vi "UDP Thread Settings UI.vi"(8 "error in (no error)":errorcluster, 10 "User Interface Events":refnum<class "User Interface Events.lvclass">, 11 "Configuration in":refnum<class "Configuration.lvclass">) -> (0 "error out":errorcluster, 3 "Configuration out":refnum<class "Configuration.lvclass">)   [LabVIEW 2017, in "DSF Core.lvlib"]
uses:
  DSF Core.lvlib
  Classes/Configuration/Configuration.lvclass
  Classes/User Interface Events/User Interface Events.lvclass
  Configuration/DSF UDP Thread Settings.lvclass
  C:/Git/DSF/Core/Classes/Configuration/Configuration.lvclass
panel:
  in  "local port":u16
  in  "local address":string
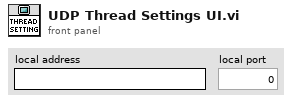
[diagram p1: front panel]
types:
  T1 = typedef "DSF Core.lvlib/DSF UDP Thread Settings.lvclass/Thread Settings.ctl" = cluster{"local port":u16, "local address":u32}
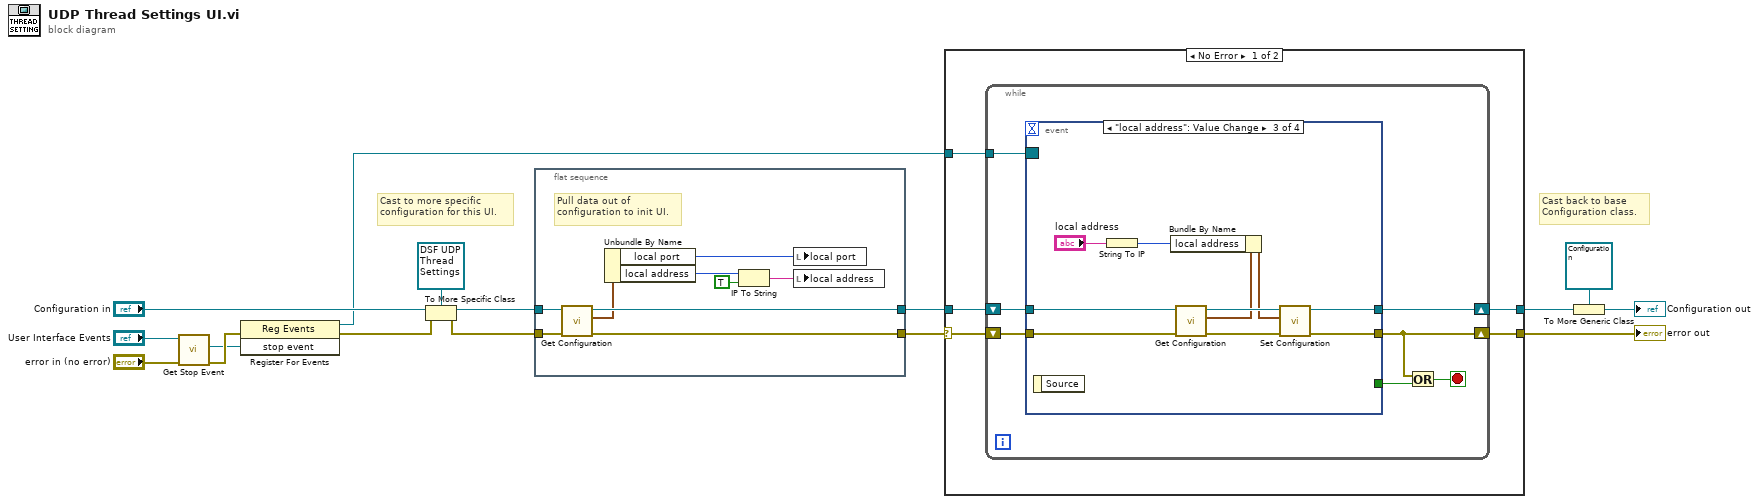
[diagram p0: block diagram]
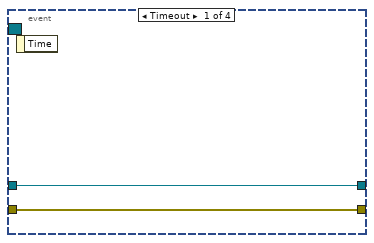
[diagram p2: hidden frame]
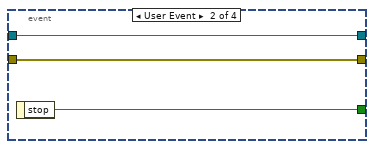
[diagram p3: hidden frame]
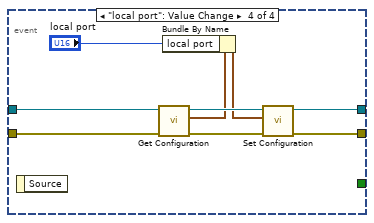
[diagram p4: hidden frame]
diagram:
  # "Cast back to base Configuration class."
  # "Cast to more specific configuration for this UI."
  n1 = call "Get Stop Event.vi"("error in (no error)"="error in (no error)", "User Interface Events in"="User Interface Events") -> ("error out"=w5:errorcluster, "stop event"=w3:refnum<user-event>)  [unwired: 7 in, 1 out]
  n2 = register-events(error in=w5, w3) -> (reference out=w6:refnum<event-registration>, error out=w7:errorcluster)  [unwired: 1 in]
  n3 = To More Specific Class(target class=refnum<class "DSF UDP Thread Settings.lvclass"> refnum ("DSF Core.lvlib:DSF UDP Thread Configuration"), reference="Configuration in", error in=w7) -> (specific class reference=w10:refnum<class "DSF UDP Thread Settings.lvclass">, error out=w11:errorcluster)
  n4 = flat-sequence {
    tunnel: [w21] -> w2
    tunnel: w11 -> [w23]
    tunnel: w10 -> [w22]
    tunnel: [w20] -> w9
    frame #0 {
      # "Pull data out of configuration to init UI."
      n5 = call "Get Configuration.vi"("error in (no error)"=w23, "DSF UDP Thread Configuration in"=w22) -> ("error out"=w21:errorcluster, "thread settings"=w19:T1, "DSF UDP Thread Configuration out"=w20:refnum<class "DSF UDP Thread Settings.lvclass">)  [unwired: 7 in]
      n6 = Unbundle By Name(w19) -> ("local port"=w17:u16, "local address"=w25:u32)
      n7 = IP To String(1:TRUE ("dot notation? (F)"), 2:w25) -> (0:w18:string)
      n8 = local write "local port"(w17) -> ()
      n9 = local write "local address"(w18) -> ()
    }
  }
  n10 = case shown="No Error" w2 {
    selector: w2 -> [w26 w62]
    tunnel: w6 -> [w30 _]
    tunnel: w9 -> [w29 w63]
    tunnel: [w28 w63] -> w15
    tunnel: [w27 w62] -> w14
    frame No Error {
      n11 = while {
        tunnel: w30 -> [w37]
        shift-right: [w35] -> w27
        shift-left: w26 -> [w36]
        shift-right: [w31] -> w28
        shift-left: w29 -> [w32]
        stop <- w34 stop-if-true
        n12 = event shown="[2] \"local address\": Value Change" {
          selector: w37 -> [_ _ _ _]
          dyn-events: _ -> [_ _ _ _]
          timeout: _ -> [_ _ _ _]
          tunnel: [_ w40 _ _] -> w33
          tunnel: w36 -> [w39 w42 w52 w61]
          tunnel: [w39 w42 w48 w57] -> w35
          tunnel: w32 -> [w38 w41 w51 w60]
          tunnel: [w38 w41 w47 w56] -> w31
          event Timeout {
            n13 = event-data() -> ()  [unwired: 1 in, 1 out]
          }
          event User Event {
            n14 = event-data() -> ("stop"=w40:bool)  [unwired: 1 in]
          }
          event "local address": Value Change {
            n15 = event-data() -> ()  [unwired: 1 in, 1 out]
            n16 = String To IP(1:"local address") -> (0:w43:u32)
            n17 = call "Get Configuration.vi"("error in (no error)"=w52, "DSF UDP Thread Configuration in"=w51) -> ("error out"=w49:errorcluster, "thread settings"=w46:T1, "DSF UDP Thread Configuration out"=w50:refnum<class "DSF UDP Thread Settings.lvclass">)  [unwired: 7 in]
            n18 = Bundle By Name(cluster=w46, "local address"=w43) -> (w45:T1)
            n19 = call "Set Configuration.vi"("error in (no error)"=w49, "thread settings"=w45, "DSF UDP Thread Configuration in"=w50) -> ("error out"=w48:errorcluster, "DSF UDP Thread Configuration out"=w47:refnum<class "DSF UDP Thread Settings.lvclass">)  [unwired: 7 in]
          }
          event "local port": Value Change {
            n20 = event-data() -> ()  [unwired: 1 in, 1 out]
            n21 = call "Get Configuration.vi"("error in (no error)"=w61, "DSF UDP Thread Configuration in"=w60) -> ("error out"=w58:errorcluster, "thread settings"=w55:T1, "DSF UDP Thread Configuration out"=w59:refnum<class "DSF UDP Thread Settings.lvclass">)  [unwired: 7 in]
            n22 = Bundle By Name(cluster=w55, "local port"="local port") -> (w54:T1)
            n23 = call "Set Configuration.vi"("error in (no error)"=w58, "thread settings"=w54, "DSF UDP Thread Configuration in"=w59) -> ("error out"=w57:errorcluster, "DSF UDP Thread Configuration out"=w56:refnum<class "DSF UDP Thread Settings.lvclass">)  [unwired: 7 in]
          }
        }
        n24 = Or(x=w35, y=w33) -> (x .or. y?=w34:bool)
      }
    }
    frame Error {
    }
  }
  "error out" <- w14
  n25 = To More Generic Class(target class=refnum<class "Configuration.lvclass"> refnum ("Configuration out"), reference=w15) -> (generic class reference=→"Configuration out":refnum<class "Configuration.lvclass">)
